vi "Gauss Function (obs).vi"(4 "c":dbl format="%.2f", 5 "b":dbl format="%.2f", 6 "a":dbl format="%.2f", 7 "x":dbl format="%.2f") -> (3 "F(x, a, b, c)":dbl format="%.2f")   [LabVIEW 2014, in "NI_Gmath.lvlib"]
doc: "Computes the Gauss hypergeometric function <B>F(x, a, b, c)</B> according to the input argument and parameters you specify."
uses:
  NI_Gmath.lvlib
  lvanlys.dll
panel:
  # "This VI is obsolete !!!\nYou should replace this VI in your diagram with the \nGauss Function VI."
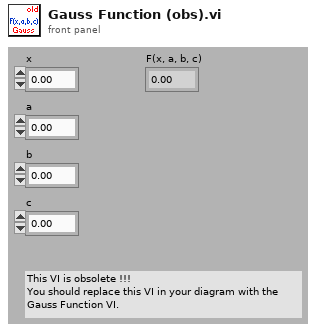
[diagram p1: front panel]
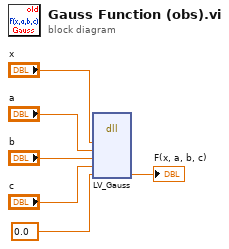
[diagram p0: block diagram]
diagram:
  n1 = dll-call lib="C:/Program Files (x86)/National Instruments/LabVIEW 2014/resource/lvanlys.*" fn="LV_Gauss"("x"="x", "a"="a", "b"="b", "c"="c", "Gauss(x, a, b, c)"=0.0 ("Gauss")) -> ("Gauss(x, a, b, c)"=→"F(x, a, b, c)":dbl)  [unwired: 8 in, 2 out]
